vi "Load Tables.vi"(1 "Error In":errorcluster) -> (0 "Error Out":errorcluster)   [LabVIEW 2018]
uses:
  Type Defs/RT Command.ctl
  Type Defs/Global Action.ctl
  <vilib>/Utility/config.llb/Write Key (String).vi
  <vilib>/Utility/config.llb/Read Key (String).vi
  <vilib>/Utility/config.llb/NI_LVConfig.lvlib
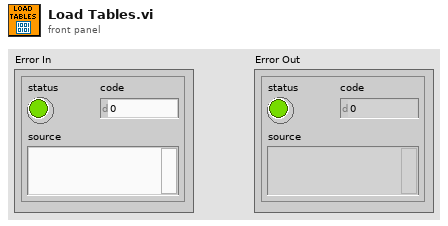
[diagram p1: front panel]
types:
  T1 = typedef "Global Action.ctl" = enum16{"Write", "Read"}
  T2 = typedef "RT Command.ctl" = enum16{"xml Start Run", "xml Start Actual Run", "xml Stop Run", "xml Runtime Update", "xml Get Status", "xml Get Table", "xml Set Table", "xml Get Configuration", "xml System Status", "xml Set LC Input Logic", "xml Get Data", "xml Get Info", "Start", "StartActualRun", "Stop", "Runtime Update", "Get Data", "Get Info", "Get Status", "Get Param", "Get Config", "Get Table", "Read ADC", "Set Oscillator", "Update Config", "Update Table", "Set All Pol", "Set Pol and DC", "Set Max Mass", "Toggle RP", "Toggle EL", "Set PIC", "Initialize Turbo", "Send Turbo Comm", "Close Turbo", "P1", "P2", "P3", "Send Serial", "Set LC Out", "Get LC In", "Read VAC", "Test Table", "Toggle Power", "Get Startup", "Set Startup", "Get ADC Table", "Set ADC Table", "Get Brief Status", "Get Detail Status", "Auxiliary Update", "Set CC Logics", "Set CC Input Logics", "Ignore Error", "invalid"}
  T3 = typedef "NI_LVConfig.lvlib/Config Data RefNum.ctl" = refnum<k1>
  T4 = typedef "Global Parameters.ctl" = cluster{"Calibrations":cluster{"Q1 +ve":dbl[][], "Q2 +ve":dbl[][], "Q1 -ve":dbl[][], "Q2 -ve":dbl[][]}, "Resolution Q1":cluster{"High +ve":dbl[][], "Med +ve":dbl[][], "Low +ve":dbl[][], "High -ve":dbl[][], "Med -ve":dbl[][], "Low -ve":dbl[][]}, "Resolution Q2":cluster{"High +ve":dbl[][], "Med +ve":dbl[][], "Loe +ve":dbl[][], "High -ve":dbl[][], "Med -ve":dbl[][], "Low -ve":dbl[][]}, "MR Parameters":T5, "Mass":dbl[][], "Dwell":dbl[][], "Steps":i32[][], "Method Refnum":refnum<vi>}
  T5 = typedef "MR Parameters.ctl" = cluster{"Name":string, "Ch#":u8, "StartV":dbl, "StopV":dbl, "StepV":dbl, "Index":u8}
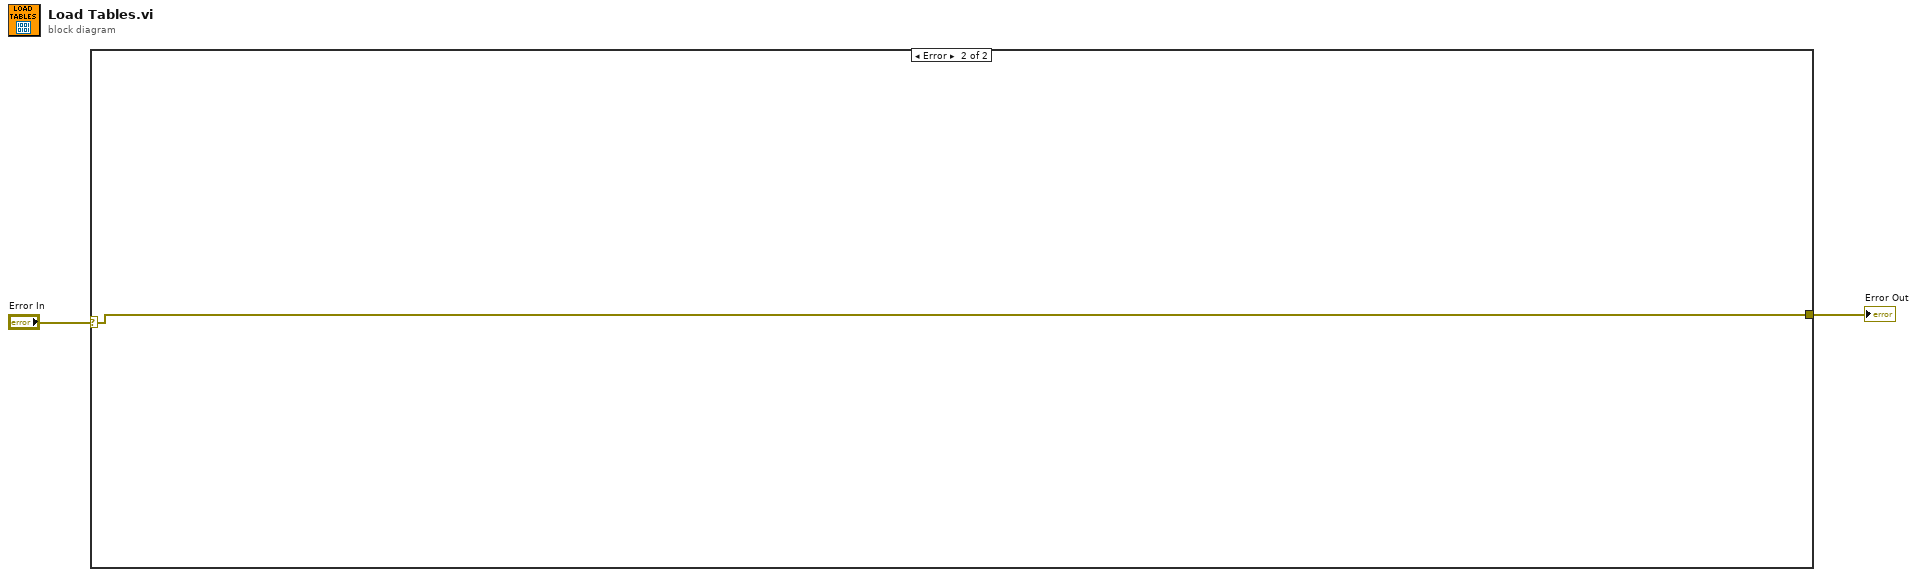
[diagram p0: block diagram]
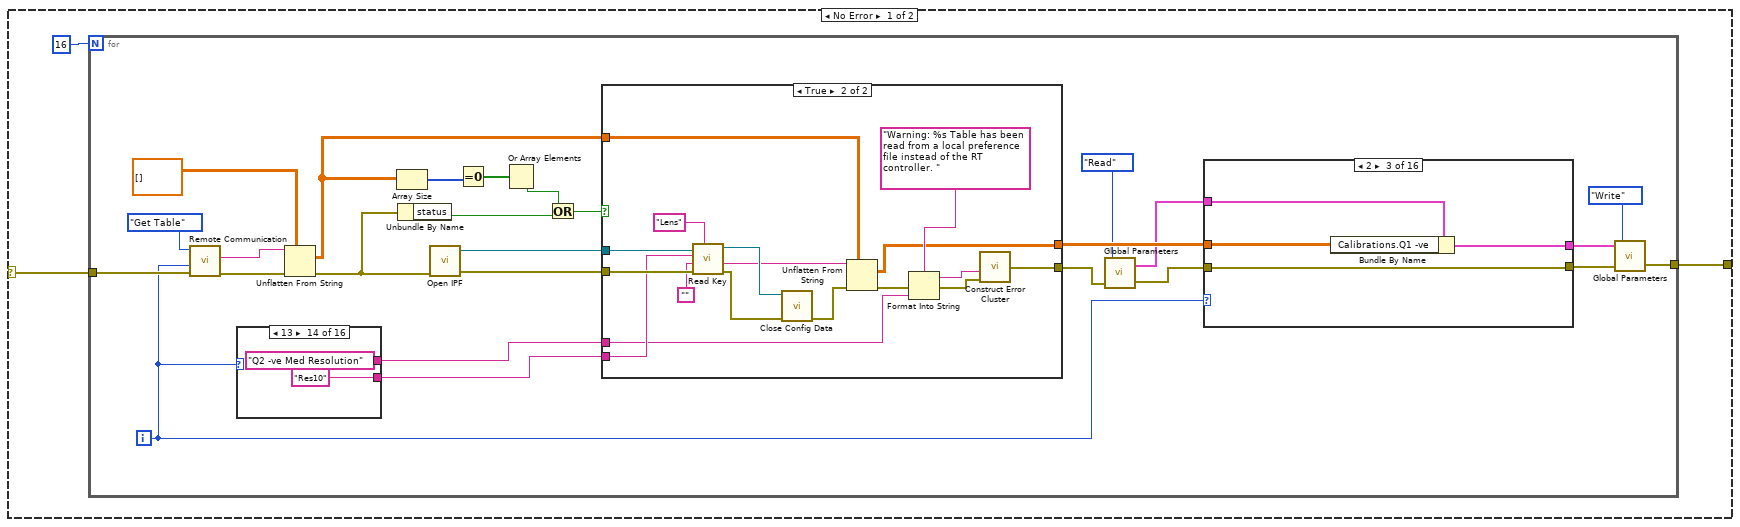
[diagram p2: hidden frame]
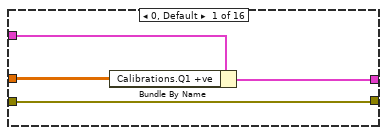
[diagram p3: hidden frame]
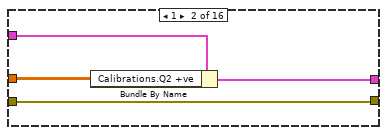
[diagram p4: hidden frame]
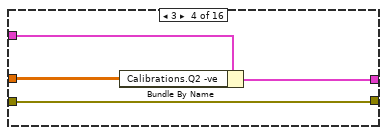
[diagram p5: hidden frame]
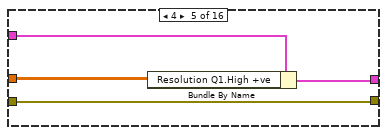
[diagram p6: hidden frame]
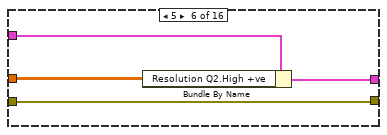
[diagram p7: hidden frame]
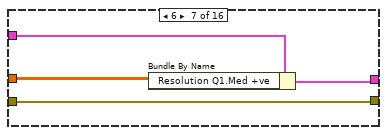
[diagram p8: hidden frame]
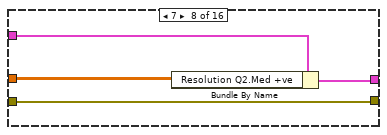
[diagram p9: hidden frame]
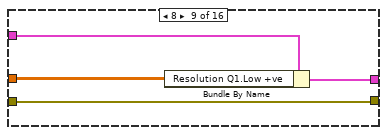
[diagram p10: hidden frame]
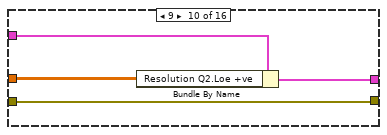
[diagram p11: hidden frame]
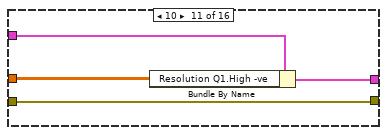
[diagram p12: hidden frame]
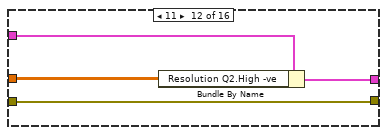
[diagram p13: hidden frame]
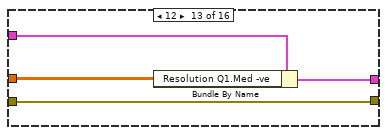
[diagram p14: hidden frame]
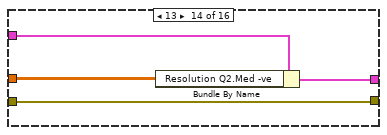
[diagram p15: hidden frame]
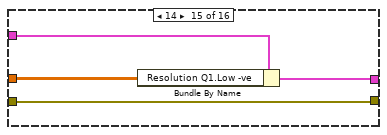
[diagram p16: hidden frame]
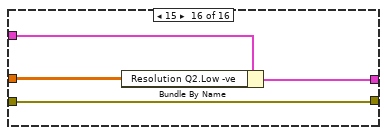
[diagram p17: hidden frame]
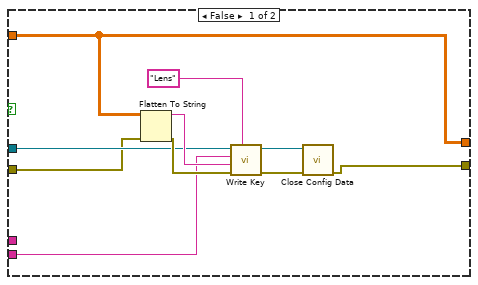
[diagram p18: hidden frame]
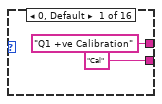
[diagram p19: hidden frame]
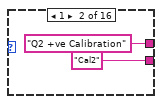
[diagram p20: hidden frame]
diagram:
  n1 = case shown="Error" "Error In" {
    selector: "Error In" -> [w4 w155]
    tunnel: [w3 w155] -> w1
    frame No Error {
      n2 = for {
        N: 16 -> [_]
        tunnel: w4 -> [w31]
        tunnel: [w11] -> w3
        i -> [w15]
        n3 = call "Remote Communication.vi"("Error In"=w31, "DC Param"=w15, "Command"=RT_Command."Get Table") -> ("Error Out"=w25:errorcluster, "Info"=w29:string)  [unwired: 3 in, 2 out]
        n4 = case shown="13" w15 {
          tunnel: ["Q1 +ve Calibration" ("section") "Q2 +ve Calibration" ("section") "Q1 -ve Calibration" ("section") "Q2 -ve Calibration" ("section") "Q1 +ve Hi Resolution" ("section") "Q2 +ve Hi Resolution" ("section") "Q1 +ve Med Resolution" ("section") "Q2 +ve Med Resolution" ("section") "Q1 +ve Low Resolution" ("section") "Q2 +ve Low Resolution" ("section") "Q1 -ve Hi Resolution" ("section") "Q2 -ve Hi Resolution" ("section") "Q1 -ve Med Resolution" ("section") "Q2 -ve Med Resolution" ("section") "Q1 -ve Low Resolution" ("section") "Q2 -ve Low Resolution" ("section")] -> w16
          tunnel: ["Cal" ("section") "Cal2" ("section") "Cal3" ("section") "Cal4" ("section") "Res" ("section") "Res2" ("section") "Res3" ("section") "Res4" ("section") "Res5" ("section") "Res6" ("section") "Res7" ("section") "Res8" ("section") "Res9" ("section") "Res10" ("section") "Res11" ("section") "Res12" ("section")] -> w17
          frame 0, Default {
          }
          frame 1 {
          }
          frame 2 {
          }
          frame 3 {
          }
          frame 4 {
          }
          frame 5 {
          }
          frame 6 {
          }
          frame 7 {
          }
          frame 8 {
          }
          frame 9 {
          }
          frame 10 {
          }
          frame 11 {
          }
          frame 12 {
          }
          frame 13 {
          }
          frame 14 {
          }
          frame 15 {
          }
        }
        n5 = Unflatten From String(type=dbl[][] [] ("Cal-"), binary string=w29, error in (no error)=w25) -> (value=w20:dbl[][], error out=w22:errorcluster)  [unwired: 3 out]
        n6 = Array Size(array=w20) -> (size(s)=w27:i32[])
        n7 = Unbundle By Name(w22) -> ("status"=w23:bool)
        n8 = call "Open IPF.vi"("Error In"=w22) -> ("Error Out"=w19:errorcluster, "IPF refnum"=w18:T3)  [unwired: 2 in, 1 out]
        n9 = Equal To 0?(x=w27) -> (x = 0?=w24:bool[])
        n10 = Or Array Elements(Boolean array=w24) -> (logical OR=w26:bool)
        n11 = Or(x=w26, y=w23) -> (x .or. y?=w21:bool)
        n12 = case shown="True" w21 {
          tunnel: w20 -> [w102 w116]
          tunnel: w19 -> [w101 w122]
          tunnel: w18 -> [w103 w121]
          tunnel: w17 -> [w96 w119]
          tunnel: w16 -> [_ w115]
          tunnel: [w98 w107] -> w8
          tunnel: [w102 w106] -> w14
          frame False {
            n13 = Flatten To String(anything=w102, error in (no error)=w101) -> (data string=w105:string, error out=w104:errorcluster)  [unwired: 3 out]
            n14 = call-poly <vilib>:"Write Key.vi"("section"="Lens", "error in (no error)"=w104, "value"=w105, "key"=w96, "refnum"=w103) -> ("error out"=w100:errorcluster, "refnum out"=w99:T3)  [unwired: 1 in, 4 out]
            n15 = call <vilib>:"Close Config Data.vi"("error in (no error)"=w100, "refnum"=w99) -> ("error out"=w98:errorcluster)  [unwired: 8 in, 1 out]
          }
          frame True {
            n16 = call-poly <vilib>:"Read Key.vi"("section"="Lens", "error in (no error)"=w122, "default value"="", "key"=w119, "refnum"=w121) -> ("error out"=w113:errorcluster, "value"=w111:string, "refnum out"=w112:T3)  [unwired: 1 in, 3 out]
            n17 = call <vilib>:"Close Config Data.vi"("error in (no error)"=w113, "refnum"=w112) -> ("error out"=w110:errorcluster)  [unwired: 8 in, 1 out]
            n18 = Unflatten From String(type=w116, binary string=w111, error in (no error)=w110) -> (value=w106:dbl[][], error out=w114:errorcluster)  [unwired: 3 out]
            n19 = Format Into String(format string="Warning: %s Table has been read from a local preference file instead of the RT controller. ", error in=w114, w115) -> (resulting string=w109:string, error out=w108:errorcluster)  [unwired: 1 in]
            n20 = call "Construct Error Cluster.vi"("Error In"=w108, "Reason"=w109) -> ("Error Out"=w107:errorcluster)  [unwired: 2 in]
          }
        }
        n21 = call "Global Parameters.vi"("Error In"=w8, "Action"=Global_Action."Read") -> ("Error Out"=w7:errorcluster, "Parameters Out"=w6:T4)  [unwired: 1 in]
        n22 = case shown="2" w15 {
          tunnel: w14 -> [w32 w39 w41 w44 w50 w54 w57 w61 w65 w69 w73 w77 w81 w85 w89 w94]
          tunnel: [w33 w38 w42 w46 w51 w55 w58 w62 w67 w71 w75 w79 w82 w87 w91 w95] -> w13
          tunnel: w7 -> [w34 w37 w40 w45 w48 w52 w56 w60 w64 w68 w72 w76 w80 w84 w88 w93]
          tunnel: [w34 w37 w40 w45 w48 w52 w56 w60 w64 w68 w72 w76 w80 w84 w88 w93] -> w12
          tunnel: w6 -> [w35 w36 w43 w47 w49 w53 w59 w63 w66 w70 w74 w78 w83 w86 w90 w92]
          frame 0, Default {
            n23 = Bundle By Name(cluster=w35, "Calibrations.Q1 +ve"=w32) -> (w33:T4)
          }
          frame 1 {
            n24 = Bundle By Name(cluster=w36, "Calibrations.Q2 +ve"=w39) -> (w38:T4)
          }
          frame 2 {
            n25 = Bundle By Name(cluster=w43, "Calibrations.Q1 -ve"=w41) -> (w42:T4)
          }
          frame 3 {
            n26 = Bundle By Name(cluster=w47, "Calibrations.Q2 -ve"=w44) -> (w46:T4)
          }
          frame 4 {
            n27 = Bundle By Name(cluster=w49, "Resolution Q1.High +ve"=w50) -> (w51:T4)
          }
          frame 5 {
            n28 = Bundle By Name(cluster=w53, "Resolution Q2.High +ve"=w54) -> (w55:T4)
          }
          frame 6 {
            n29 = Bundle By Name(cluster=w59, "Resolution Q1.Med +ve"=w57) -> (w58:T4)
          }
          frame 7 {
            n30 = Bundle By Name(cluster=w63, "Resolution Q2.Med +ve"=w61) -> (w62:T4)
          }
          frame 8 {
            n31 = Bundle By Name(cluster=w66, "Resolution Q1.Low +ve"=w65) -> (w67:T4)
          }
          frame 9 {
            n32 = Bundle By Name(cluster=w70, "Resolution Q2.Loe +ve"=w69) -> (w71:T4)
          }
          frame 10 {
            n33 = Bundle By Name(cluster=w74, "Resolution Q1.High -ve"=w73) -> (w75:T4)
          }
          frame 11 {
            n34 = Bundle By Name(cluster=w78, "Resolution Q2.High -ve"=w77) -> (w79:T4)
          }
          frame 12 {
            n35 = Bundle By Name(cluster=w83, "Resolution Q1.Med -ve"=w81) -> (w82:T4)
          }
          frame 13 {
            n36 = Bundle By Name(cluster=w86, "Resolution Q2.Med -ve"=w85) -> (w87:T4)
          }
          frame 14 {
            n37 = Bundle By Name(cluster=w90, "Resolution Q1.Low -ve"=w89) -> (w91:T4)
          }
          frame 15 {
            n38 = Bundle By Name(cluster=w92, "Resolution Q2.Low -ve"=w94) -> (w95:T4)
          }
        }
        n39 = call "Global Parameters.vi"("Error In"=w12, "Action"=Global_Action."Write", "Parameters In"=w13) -> ("Error Out"=w11:errorcluster)  [unwired: 1 out]
      }
    }
    frame Error {
    }
  }
  "Error Out" <- w1
